vi "choosePositionForDefender.vi"(6 "Robot":refnum<class "Robot.lvclass">, 8 "error in (no error)":errorcluster, 9 "Odered array of robots":dbl[][](array[numeric]), 10 "Ordered Positions To Go":dbl[][](array[numeric]), 11 "DefendAreaSkill in":refnum<class "DefendAreaSkill.lvclass">) -> (0 "error out":errorcluster, 2 "Position":dbl[](array[numeric]), 3 "DefendAreaSkill out":refnum<class "DefendAreaSkill.lvclass">)   [LabVIEW 2024, in "DefendAreaSkill.lvclass"]
uses:
  DefendAreaSkill.lvclass
  Robot_class/Robot.lvclass
  Robot_class/Robot.lvclass/Robot.ctl
  Robot_class/Read id.vi
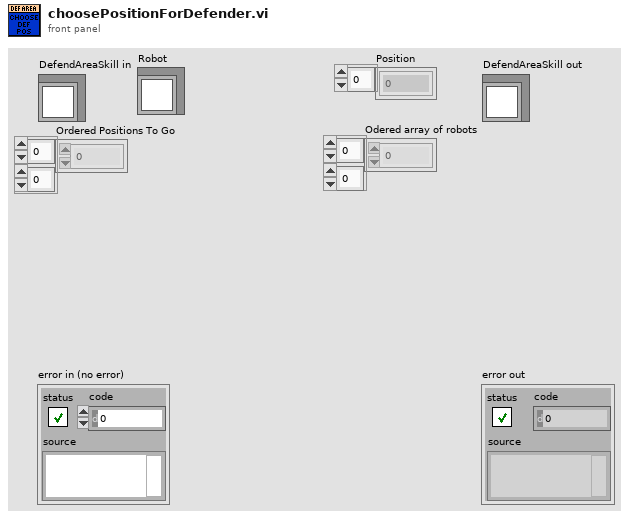
[diagram p1: front panel]
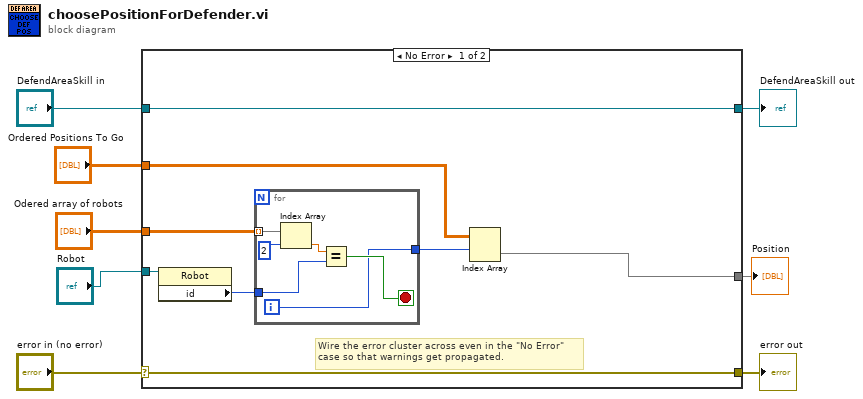
[diagram p0: block diagram]
diagram:
  n1 = case shown="No Error" "error in (no error)" {
    selector: "error in (no error)" -> [w15 w24]
    tunnel: [w15 w24] -> w7
    tunnel: [w16 w23] -> w5
    tunnel: "DefendAreaSkill in" -> [w16 w23]
    tunnel: "Odered array of robots" -> [w14 _]
    tunnel: "Robot" -> [w13 _]
    tunnel: "Ordered Positions To Go" -> [w10 _]
    tunnel: [w9 _] -> w1
    frame No Error {
      # "Wire the error cluster across even in the \"No Error\"\ncase so that warnings get propagated."
      n2 = property class="Robot"(reference=w13) -> ("id"=w12:i32)  [unwired: 1 in, 2 out]
      n3 = for {
        tunnel: w14 -> [w22] mode=indexing
        tunnel: w12 -> [w19]
        tunnel: [w17] -> w11
        i -> [w17]
        stop <- w18 stop-if-true
        n4 = Index Array(array=w22, index=2) -> (element=w20:dbl)
        n5 = Equal?(x=w20, y=w19) -> (x = y?=w18:bool)
      }
      n6 = Index Array(array=w10, index (row)=w11) -> (element=w9:dbl[])  [unwired: 1 in]
    }
    frame Error {
    }
  }
  "error out" <- w7
  "DefendAreaSkill out" <- w5
  "Position" <- w1
